vi "Practica2_Tipos de datos.vi"() -> ()   [LabVIEW 2022 SP3]
panel:
  out "Path 2":path
  in  "Path":path
  out "Ring 2":u16(ring)
  in  "Ring":u16(ring)
  out "Cluster 2":T1 {"Meter" scale=0.0..10.0; "Slide" scale=0.0..50.0}
  in  "Cluster":T2 {"Slide" scale=0.0..10.0; "Dial" scale=0.0..50.0}
  in  "Array 2":bool[](array[boolean])
  out "Array":bool[](array[boolean])
  out "Combo Box 2":string(combo)
  in  "Combo Box":string(combo)
  out "String 2":string
  in  "String":string
  out "Boolean 2":bool
  in  "Boolean":bool
  out "Numeric 6":dbl
  in  "Numeric 5":dbl
  out "Numeric 4":dbl
  in  "Numeric 3":dbl
  out "Numeric 2":dbl
  in  "Numeric":dbl
  # "Anahí Montserrat Vázquez Padilla \nPráctica 02: Tipos de datos\n24/01/2024"
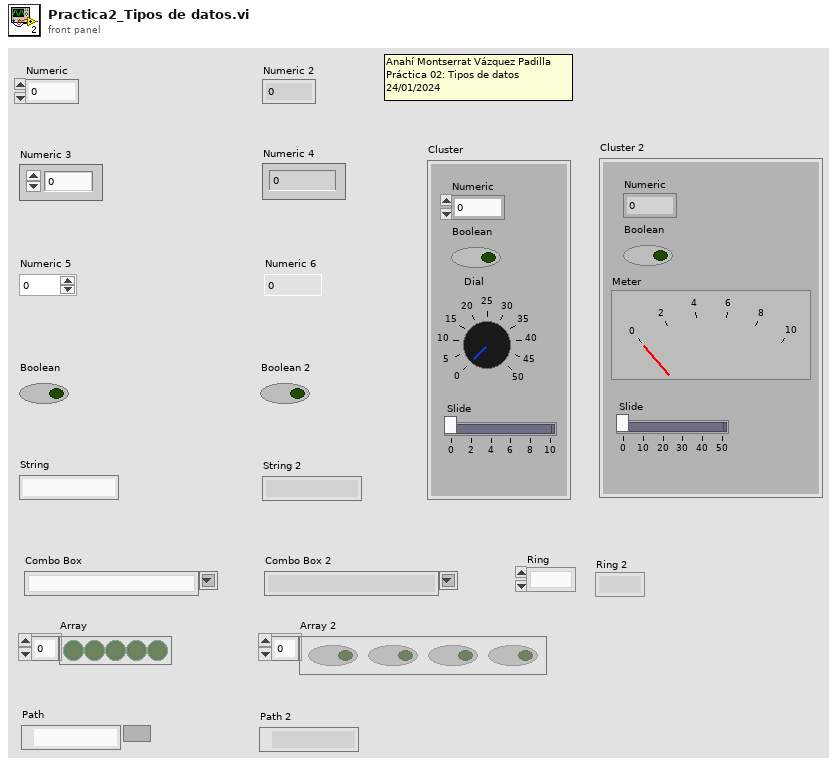
[diagram p1: front panel]
types:
  T1 = cluster{"Numeric":dbl, "Boolean":bool, "Slide":dbl, "Meter":dbl}
  T2 = cluster{"Numeric":dbl, "Boolean":bool, "Dial":dbl, "Slide":dbl}
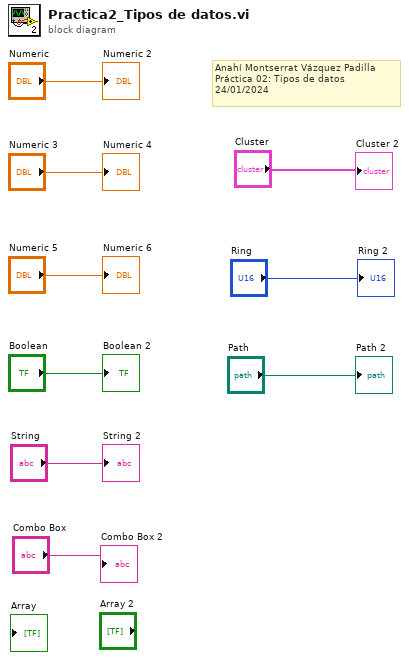
[diagram p0: block diagram]
diagram:
  # "Anahí Montserrat Vázquez Padilla \nPráctica 02: Tipos de datos\n24/01/2024"
  "Numeric 2" <- "Numeric"
  "Numeric 4" <- "Numeric 3"
  "Numeric 6" <- "Numeric 5"
  "Boolean 2" <- "Boolean"
  "String 2" <- "String"
  "Combo Box 2" <- "Combo Box"
  "Cluster 2" <- "Cluster"
  "Ring 2" <- "Ring"
  "Path 2" <- "Path"
